vi "Create.vi"(8 "error in (no error)":errorcluster, 9 "Amount":dbl, 10 "Category Name":string, 11 "WhichMonth.lvclass":refnum<class "WhichMonth.lvclass">) -> (0 "error out":errorcluster, 3 "Goal out":refnum<class "Goal.lvclass">)   [LabVIEW 2018, in "Goal.lvclass"]
uses:
  Goal.lvclass
  C:/GitRepos/Filthy-Lucre-Budgetizer/source/support/classes/Category/Category.lvclass
  WhichMonth/WhichMonth.lvclass
  Goal.lvclass/Goal.ctl
  Category/Category.lvclass
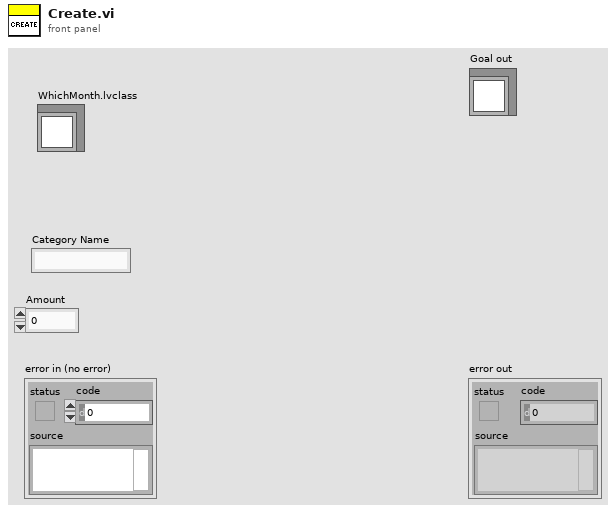
[diagram p1: front panel]
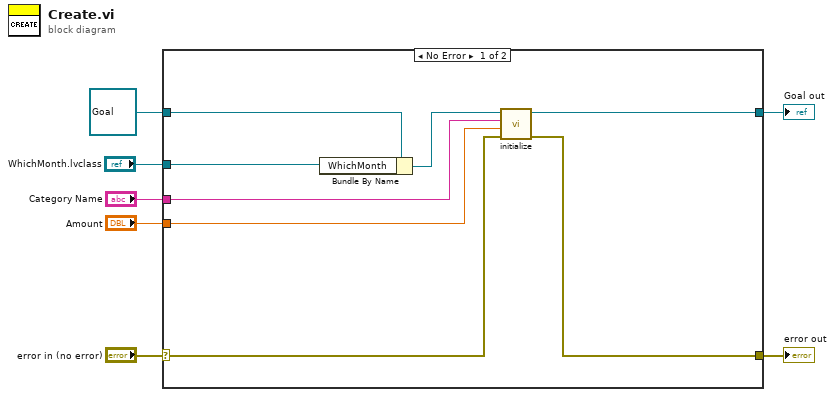
[diagram p0: block diagram]
diagram:
  n1 = case shown="No Error" "error in (no error)" {
    selector: "error in (no error)" -> [w14 w17]
    tunnel: [w13 w17] -> w6
    tunnel: refnum<class "Goal.lvclass"> refnum ("Goal in") -> [w15 w16]
    tunnel: [w8 w16] -> w4
    tunnel: "Category Name" -> [w11 _]
    tunnel: "WhichMonth.lvclass" -> [w12 _]
    tunnel: "Amount" -> [w10 _]
    frame No Error {
      n2 = Bundle By Name(cluster=w15, "WhichMonth"=w12) -> (w9:refnum<class "Goal.lvclass">)
      n3 = call "initialize.vi"("error in (no error)"=w14, "Default Goal Amount"=w10, "Name"=w11, "Category"=w9) -> ("error out"=w13:errorcluster, "Category out"=w8:refnum<class "Goal.lvclass">)  [unwired: 6 in]
    }
    frame Error {
    }
  }
  "error out" <- w6
  "Goal out" <- w4
